vi "Basic Serial Echovi.vi"(0 "VISA resource name":refnum<visa-resource-name>="COM1", 1 "baud rate":u32=9600, 2 "data bits":u16=8 min=5 max=8 step=1, 3 "parity":u16(ring) items=["None", "Odd", "Even", "Mark", "Space"], 4 "stop bits":u16(ring)=10 items=["1.0"=10, "1.5"=15, "2.0"=20], 7 "flow control":u16(ring) items=["None"=0, "XON/XOFF"=1, "RTS/CTS"=2, "DTR/DSR"=4]) -> ()   [LabVIEW 2012]
doc: "The Basic Serial Read and Write example performs a Serial Port Read, a Serial Port Write, or a combination of these actions. The user selects the actions (read or write) on the front panel. If both are selected, the VI will write the data first, read data, and then close the VISA session that is opened to the port. This VI will wait until the specified number of bytes is received at the port or until a termination character is read.\n\nINSTRUCTIONS:\n1) Select the serial resource and configuration parameters (baud rate, data bits, parity, stop bits, flow control).\n2) Select the operations to be performed. \n3) Connect the serial port to your device. If no device is available, perform a loopback test by doing one of the following. Short pins 2 and 3 on a RS-232 cable or short pin 4 to pin 8 and pin 5 to pin 9 on a RS-485/422 cable. \n4) Run the VI to see the data read. (The \"read string\" will match the \"string to write\" if a loopback test was performed.)\n\nNote: The parameters set for the serial port must match the parameters of the connected instrument or device. In this example, the bytes to read parameter specifies the number of bytes that the serial port reads. If there were more bytes at the port than the number specified in bytes to read, those bytes would not be read. Also, if you specify to read more bytes than the number of bytes actually read, you might receive a timeout error message.\n\nOn the block diagram, the Configure Serial Port VI sets the configuration parameters. The front panel displays the controls used to configure the basic parameters, such as baud rate, data bits, and parity. Constants configure the other parameters the user probably does not need set. After the VISA Configure Serial Port VI opens the VISA session and configures the port, the VI passes the VISA resource name to other VIs that perform operations on that VISA resource. The VISA Write function sends a command to the serial device and the VISA Read function returns data based on the command. The VISA Close function then closes the reference to the serial device. It is important to close the reference; otherwise communication through with that port through protocols other than VISA might not be possible."
uses:
  <vilib>/Instr/_visa.llb/VISA Configure Serial Port (Instr).vi
panel:
  out "return count":u32
  out "Bytes @ Port":u32
  in  "Echo Serial":bool
  out "String Read":string
  in  "Write Data":bool
  in  "String to Write":string
  in  "stop":bool
  in  "delay before read (ms)":u32=500
  # "On Windows/Linux, consider using the Instrument Driver Finder (Help>>Find Instrument Drivers) to search for an instrument driver for your instrument."
  # "Select the serial resource and the operations (Read, Write, or both) to be performed.  If both are selected, the VI will write the data first, read data and then close the VISA session that is opened to the port.  This VI will wait until the specified number of bytes is received at the port or until a termination character is read."
  # "For additional information select File >> VI Properties >> Documentation"
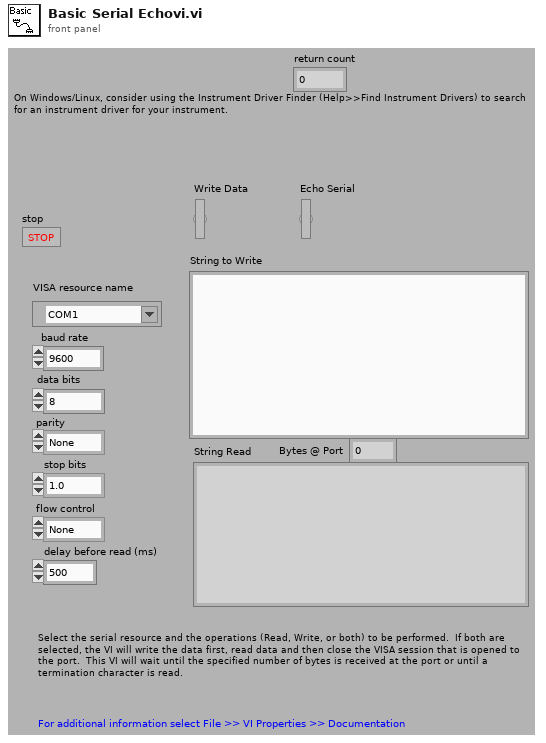
[diagram p1: front panel]
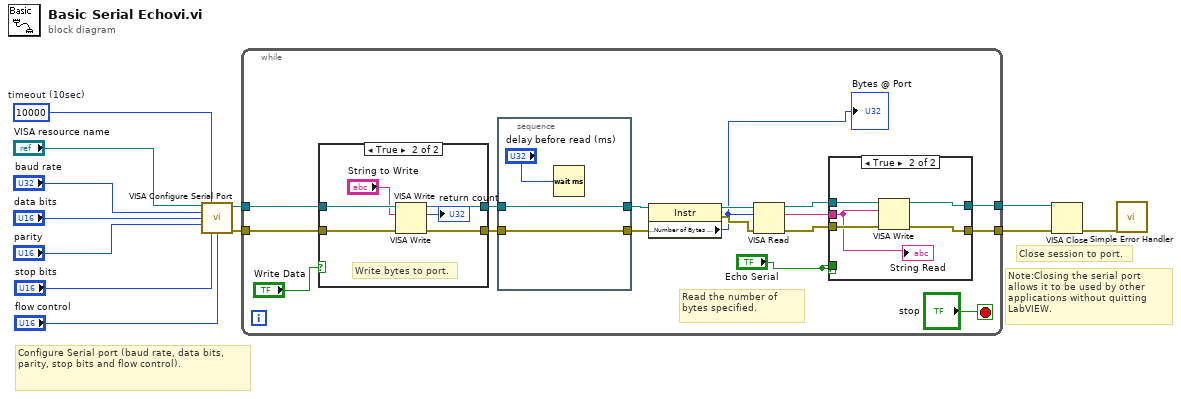
[diagram p0: block diagram]
diagram:
  w4 = u32 10000  # timeout (10sec)
  # "Note:Closing the serial port allows it to be used by other applications without quitting LabVIEW."
  # "Configure Serial port (baud rate, data bits, parity, stop bits and flow control)."
  # "Close session to port."
  n1 = call-poly "VISA Configure Serial Port"("VISA resource name"="VISA resource name", "timeout (10sec)"=w4, "baud rate (9600)"="baud rate", "data bits (8)"="data bits", "parity (0:none)"="parity", "stop bits (10: 1 bit)"="stop bits", "flow control (0:none)"="flow control") -> ("VISA resource name out"=w9:refnum<visa-resource-name>, "error out"=w10:errorcluster)  [unwired: 2 in, 5 out]
  n2 = while {
    tunnel: w10 -> [w29]
    tunnel: w9 -> [w28]
    tunnel: [w20] -> w8
    tunnel: [w21] -> w7
    stop <- "stop" stop-if-true
    # "Read the number of bytes specified."
    n3 = case shown="True" "Write Data" {
      tunnel: [w41 w44] -> w27
      tunnel: w28 -> [w40 w47]
      tunnel: w29 -> [w41 w43]
      tunnel: [w40 w45] -> w26
      frame False {
      }
      frame True {
        # "Write bytes to port."
        n4 = VISA Write(VISA resource name=w47, write buffer="String to Write", error in (no error)=w43) -> (VISA resource name out=w45:refnum<visa-resource-name>, return count=→"return count":u32, error out=w44:errorcluster)
        n5 = VISA Write() -> ()  [unwired: 3 in, 3 out]
      }
    }
    n6 = stacked-sequence {
      tunnel: w27 -> [w39]
      tunnel: [w39] -> w16
      tunnel: w26 -> [w38]
      tunnel: [w38] -> w17
      frame #0 {
        n7 = Wait (ms)(milliseconds to wait="delay before read (ms)") -> ()  [unwired: 1 out]
      }
    }
    n8 = property class="Instr"(reference=w17, error in=w16) -> (reference out=w23:refnum<visa-resource-name>, error out=w24:errorcluster, "Serial Settings:Number of Bytes at Serial Port"=w14:u32)
    "Bytes @ Port" <- w14
    n9 = VISA Read(VISA resource name=w23, byte count=w14, error in (no error)=w24) -> (VISA resource name out=w22:refnum<visa-resource-name>, read buffer=w18:string, error out=w19:errorcluster)  [unwired: 1 out]
    n10 = case shown="True" "Echo Serial" {
      tunnel: w22 -> [w31 w36]
      tunnel: [w31 w35] -> w21
      tunnel: [w30 w34] -> w20
      tunnel: w19 -> [w30 w33]
      tunnel: w18 -> [_ w32]
      tunnel: "Echo Serial" -> [_ _]
      frame False {
      }
      frame True {
        n11 = VISA Write(VISA resource name=w36, write buffer=w32, error in (no error)=w33) -> (VISA resource name out=w35:refnum<visa-resource-name>, error out=w34:errorcluster)  [unwired: 1 out]
        "String Read" <- w32
      }
    }
  }
  n12 = VISA Close(VISA resource name=w7, error in (no error)=w8) -> (error out=w6:errorcluster)
  n13 = call <vilib>:"Simple Error Handler.vi"("error in (no error)"=w6) -> ()  [unwired: 1 in, 8 out]
